vi "Set Rep Rounds.vi"(8 "error in (no error)":errorcluster, 10 "Rep Rounds":u32, 11 "Game in":refnum<class "Game.lvclass">) -> (0 "error out":errorcluster, 3 "Game out":refnum<class "Game.lvclass">)   [LabVIEW 2020, in "SquareBattle.lvlib" / "Game.lvclass"]
uses:
  Game.lvclass
  Game.lvclass/Game.ctl
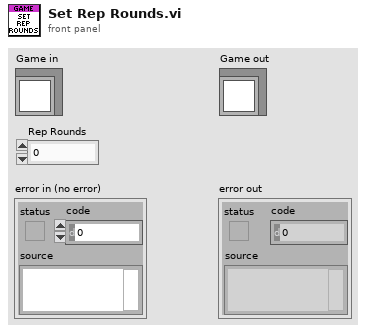
[diagram p1: front panel]
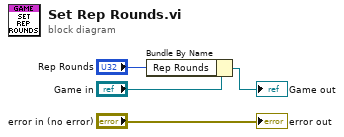
[diagram p0: block diagram]
diagram:
  n1 = Bundle By Name(cluster="Game in", "Rep Rounds"="Rep Rounds") -> (→"Game out":refnum<class "Game.lvclass">)
  "error out" <- "error in (no error)"
